vi "LF_maker2.vi"() -> ()   [LabVIEW 2014]
uses:
  <vilib>/Utility/file.llb/Read From Spreadsheet File (string).vi
  <vilib>/Utility/file.llb/Read From Spreadsheet File (I64).vi
  <vilib>/Utility/file.llb/Read From Spreadsheet File (DBL).vi
  <vilib>/Utility/file.llb/Write To Spreadsheet File (DBL).vi
panel:
  in  "피험자이름":path=path "C:/Users/Jaehong/Desktop/안전복지프로젝트/1차 2차 실험 데이터/피험자이름.txt"
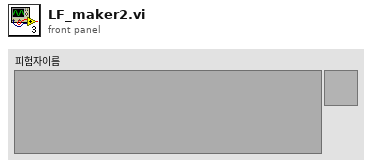
[diagram p1: front panel]
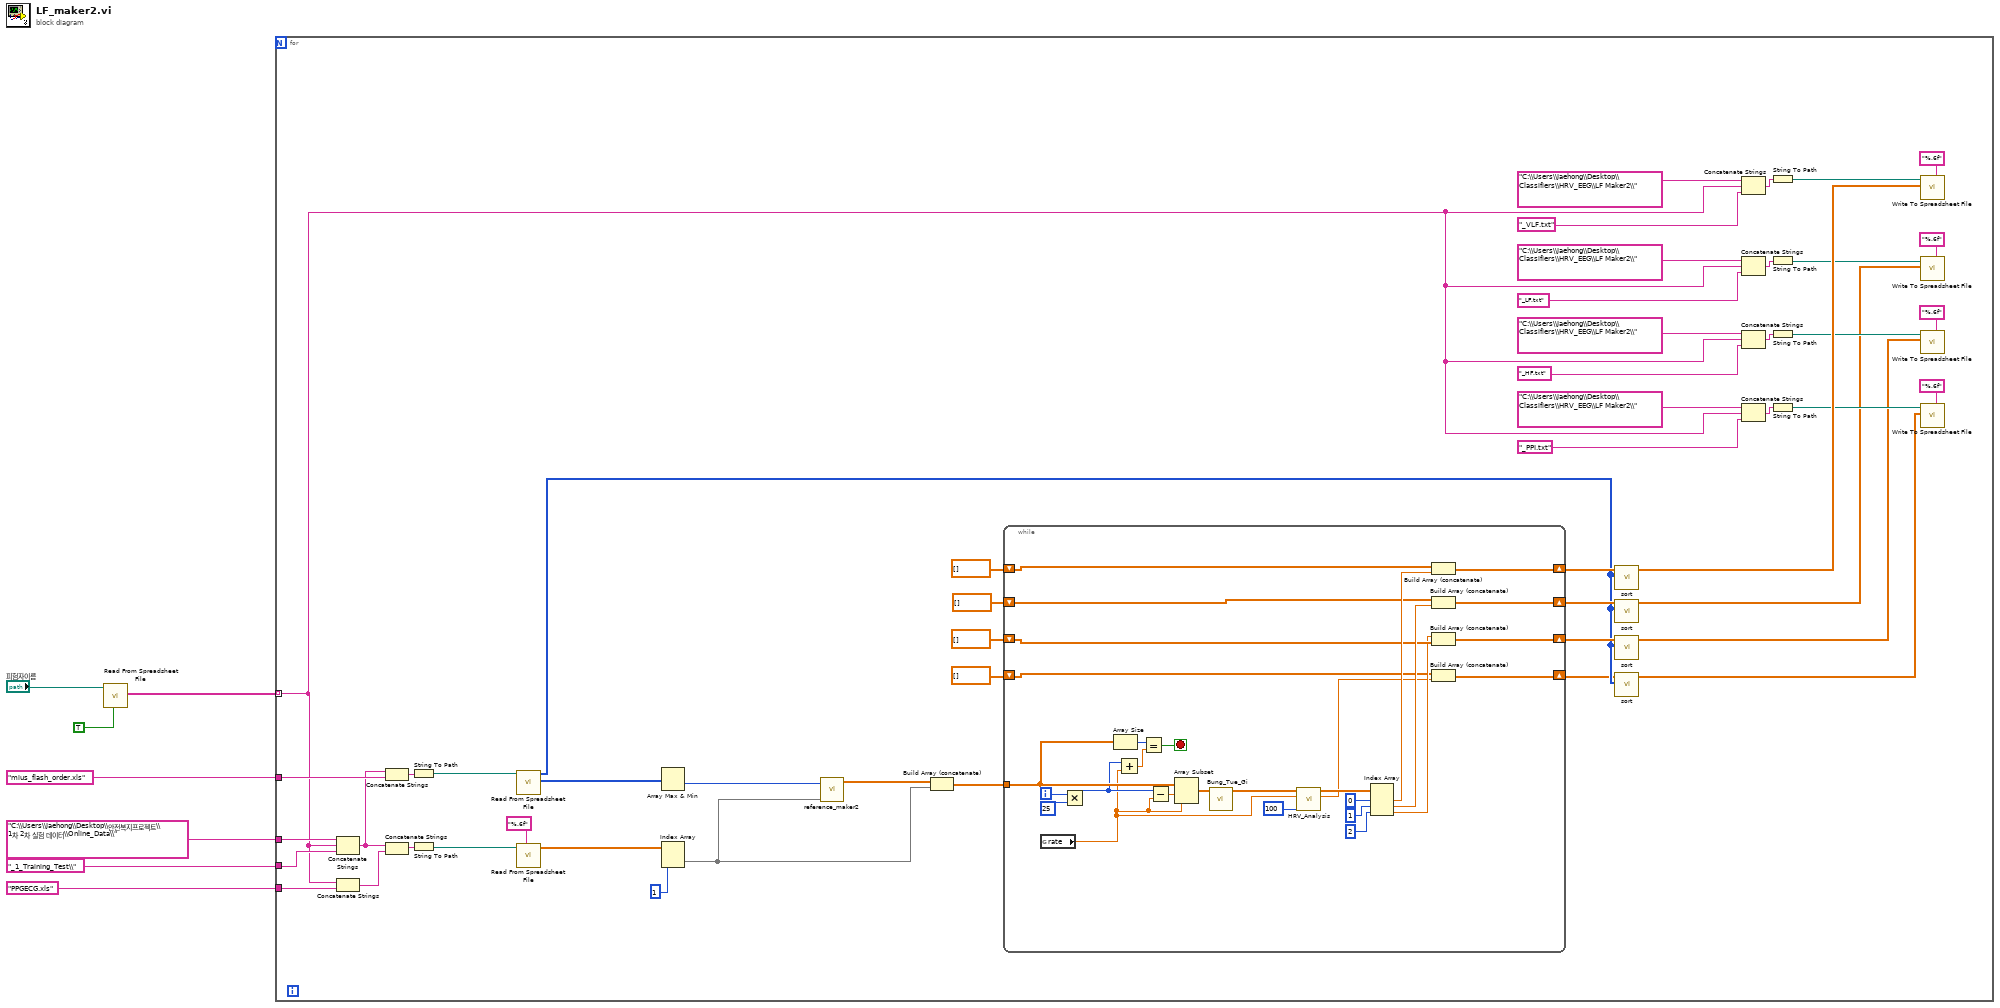
[diagram p0: block diagram]
diagram:
  n1 = call-poly <vilib>:"Read From Spreadsheet File.vi"("transpose (no:F)"=TRUE, "file path (dialog if empty)"="피험자이름") -> ("first row"=w5:string[])  [unwired: 5 in, 4 out]
  n2 = for {
    tunnel: w5 -> [w18] mode=indexing
    tunnel: "C:\\Users\\Jaehong\\Desktop\\안전복지프로젝트\\1차 2차 실험 데이터\\Online_Data\\" -> [w55]
    tunnel: "_1_Training_Test\\" -> [w54]
    tunnel: "PPGECG.xls" -> [w53]
    tunnel: "mius_flash_order.xls" -> [w50]
    n3 = Concatenate Strings(w55, w18, w54) -> (w48:string)
    n4 = Concatenate Strings(w18, w53) -> (w52:string)
    n5 = Concatenate Strings(w48, w50) -> (w49:string)
    n6 = Concatenate Strings(w48, w52) -> (w51:string)
    n7 = String To Path(string=w49) -> (path=w47:path)
    n8 = String To Path(string=w51) -> (path=w56:path)
    n9 = call-poly <vilib>:"Read From Spreadsheet File.vi"("file path (dialog if empty)"=w47) -> ("first row"=w35:i64[], "all rows"=w30:i64[][])  [unwired: 6 in, 3 out]
    n10 = call-poly <vilib>:"Read From Spreadsheet File.vi"("format (%.3f)"="%.6f", "file path (dialog if empty)"=w56) -> ("all rows"=w58:dbl[][])  [unwired: 5 in, 4 out]
    n11 = Array Max & Min(array=w35) -> (min value=w34:i64)  [unwired: 3 out]
    n12 = Index Array(array=w58, index (col)=1 ("index")) -> (element=w8:dbl[])  [unwired: 1 in]
    n13 = call "reference_maker2.vi"("Raw_PPG"=w8, "start_index"=w34) -> ("reference"=w46:dbl[])  [unwired: 9 in]
    n14 = Build Array (concatenate)(w46, w8) -> (w45:dbl[])
    n15 = while {
      tunnel: w45 -> [w87]
      shift-right: [w79] -> w33
      shift-left: dbl[] [] -> [w78]
      shift-right: [w74] -> w32
      shift-left: dbl[] [] -> [w73]
      shift-right: [w71] -> w31
      shift-left: dbl[] [] -> [w70]
      shift-right: [w68] -> w29
      shift-left: dbl[] [] -> [w66]
      i -> [w86]
      stop <- w83 stop-if-true
      n16 = global read "Control_Panel.vi" "rate"() -> (w60:dbl)
      n17 = Multiply(x=w86, y=25) -> (x*y=w65:i32)
      n18 = Array Size(array=w87) -> (size(s)=w85:i32)
      n19 = Add(x=w65, y=w60) -> (x+y=w84:dbl)
      n20 = Equal?(x=w85, y=w84) -> (x = y?=w83:bool)
      n21 = Subtract(x=w65, y=w60) -> (x-y=w61:dbl)
      n22 = Array Subset(array=w87, index=w61, length=w60) -> (w62:dbl[])
      n23 = call "Bung_Tue_Gi.vi"("Raw_PPG"=w62) -> ("reference"=w63:dbl[])  [unwired: 10 in]
      n24 = call "HRV_Analysis.vi"("Frame Length"=100, "Sample Rate"=w60, "PPG_Data"=w63) -> ("PPI"=w67:dbl, "PRV% (VLF, LF, HF)"=w81:dbl[])  [unwired: 7 in]
      n25 = Index Array(array=w81, index #1=0 ("index"), index #2=1 ("index"), index #3=2 ("index")) -> (element #1=w80:dbl, element #2=w72:dbl, element #3=w69:dbl)
      n26 = Build Array (concatenate)(w78, w80) -> (w79:dbl[])
      n27 = Build Array (concatenate)(w73, w72) -> (w74:dbl[])
      n28 = Build Array (concatenate)(w69, w70) -> (w71:dbl[])
      n29 = Build Array (concatenate)(w66, w67) -> (w68:dbl[])
    }
    n30 = call "sort.vi"("mius_flash_order"=w30, "HRV_data"=w33) -> ("appended array"=w28:dbl[][])  [unwired: 9 in]
    n31 = call "sort.vi"("mius_flash_order"=w30, "HRV_data"=w32) -> ("appended array"=w9:dbl[][])  [unwired: 9 in]
    n32 = call "sort.vi"("mius_flash_order"=w30, "HRV_data"=w31) -> ("appended array"=w10:dbl[][])  [unwired: 9 in]
    n33 = call "sort.vi"("mius_flash_order"=w30, "HRV_data"=w29) -> ("appended array"=w11:dbl[][])  [unwired: 9 in]
    n34 = Concatenate Strings("C:\\Users\\Jaehong\\Desktop\\Classifiers\\HRV_EEG\\LF Maker2\\", w18, "_VLF.txt") -> (w37:string)
    n35 = Concatenate Strings("C:\\Users\\Jaehong\\Desktop\\Classifiers\\HRV_EEG\\LF Maker2\\", w18, "_LF.txt") -> (w26:string)
    n36 = Concatenate Strings("C:\\Users\\Jaehong\\Desktop\\Classifiers\\HRV_EEG\\LF Maker2\\", w18, "_HF.txt") -> (w23:string)
    n37 = Concatenate Strings("C:\\Users\\Jaehong\\Desktop\\Classifiers\\HRV_EEG\\LF Maker2\\", w18, "_PPI.txt") -> (w20:string)
    n38 = String To Path(string=w37) -> (path=w40:path)
    n39 = String To Path(string=w26) -> (path=w16:path)
    n40 = String To Path(string=w23) -> (path=w14:path)
    n41 = String To Path(string=w20) -> (path=w12:path)
    n42 = call-poly <vilib>:"Write To Spreadsheet File.vi"("format (%.3f)"="%.6f", "2D data"=w28, "file path (dialog if empty)"=w40) -> ()  [unwired: 5 in, 1 out]
    n43 = call-poly <vilib>:"Write To Spreadsheet File.vi"("format (%.3f)"="%.6f", "2D data"=w9, "file path (dialog if empty)"=w16) -> ()  [unwired: 5 in, 1 out]
    n44 = call-poly <vilib>:"Write To Spreadsheet File.vi"("format (%.3f)"="%.6f", "2D data"=w10, "file path (dialog if empty)"=w14) -> ()  [unwired: 5 in, 1 out]
    n45 = call-poly <vilib>:"Write To Spreadsheet File.vi"("format (%.3f)"="%.6f", "2D data"=w11, "file path (dialog if empty)"=w12) -> ()  [unwired: 5 in, 1 out]
  }
